vi "Parse Auto Data.vi"(10 "Is Blue Alliance?":bool=TRUE, 11 "path":path) -> (1 "Zero Velocity?":bool[](array[boolean]), 2 "Velocities":T3[](array[typedef]), 3 "Positions":cluster{"x":dbl, "y":dbl, "th":dbl}[](array[cluster]), 5 "Commands out":cluster{"Time (s)":dbl, T1, bool}[](array[cluster]), 7 "Overall":cluster{"Time (s)":dbl, "Distance (ft)":dbl})   [LabVIEW 2023]
uses:
  swerve/Type Definitions/Data/Robot Velocities.ctl
  bordeaux-pathinator/Bordeaux/Types/Single Cmd Info.ctl
  <vilib>/picture/picture.llb/imagedata.ctl
  <vilib>/Analysis/coordinate.llb/2D Cartesian Coordinate Rotation (Scalar).vi
  <vilib>/Analysis/NI_AALPro.lvlib
panel:
  out "XY Graph":cluster{dbl[], dbl[]}[](graph)
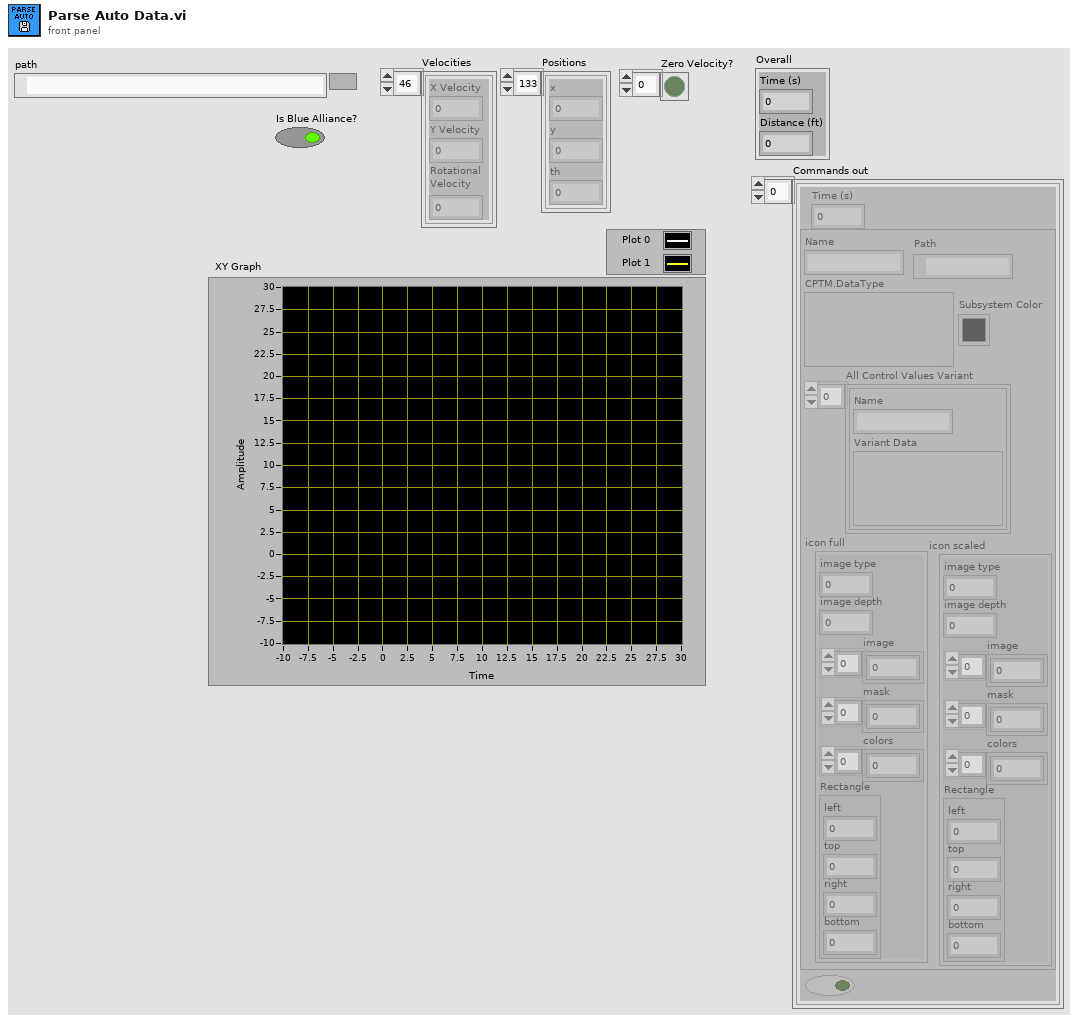
[diagram p1: front panel]
types:
  T1 = typedef "Single Cmd Info.ctl" = cluster{"Name":string, "CPTM.DataType":variant, "All Control Values Variant":cluster{"Name":string, "Variant Data":variant}[], "icon full":T2, "icon scaled":T2, "Path":path, "Subsystem Color":u32}
  T2 = typedef "imagedata.ctl" = cluster{"image type":i32, "image depth":i32, "image":u8[], "mask":u8[], "colors":u32[], "Rectangle":cluster{"left":i16, "top":i16, "right":i16, "bottom":i16}}
  T3 = typedef "Robot Velocities.ctl" = cluster{"X Velocity":dbl, "Y Velocity":dbl, "Rotational \nVelocity":dbl}
  T4 = typedef "Trajectory Data.ctl" = cluster{"Segment Name":string, "Type":T5, "Traj Pos Points":cluster{"x":dbl, "y":dbl, "th":dbl}[], "Traj Vel Points":cluster{"V":dbl, "Omega":dbl, "V vector":cluster{"y":dbl, "x":dbl}}[], "Accel Index":i32, "Decel Index":i32}[]
  T5 = typedef "Segment Type.ctl" = enum16{"Accel Straight", "Const Straight", "Blend", "Circle", "Bezier"}
  T6 = typedef "WPI_DriverStationAllianceInfo.ctl" = enum16{"Red", "Blue", "Invalid"}
  T7 = cluster{"V":dbl, "Omega":dbl, "V vector":cluster{"y":dbl, "x":dbl}}[]
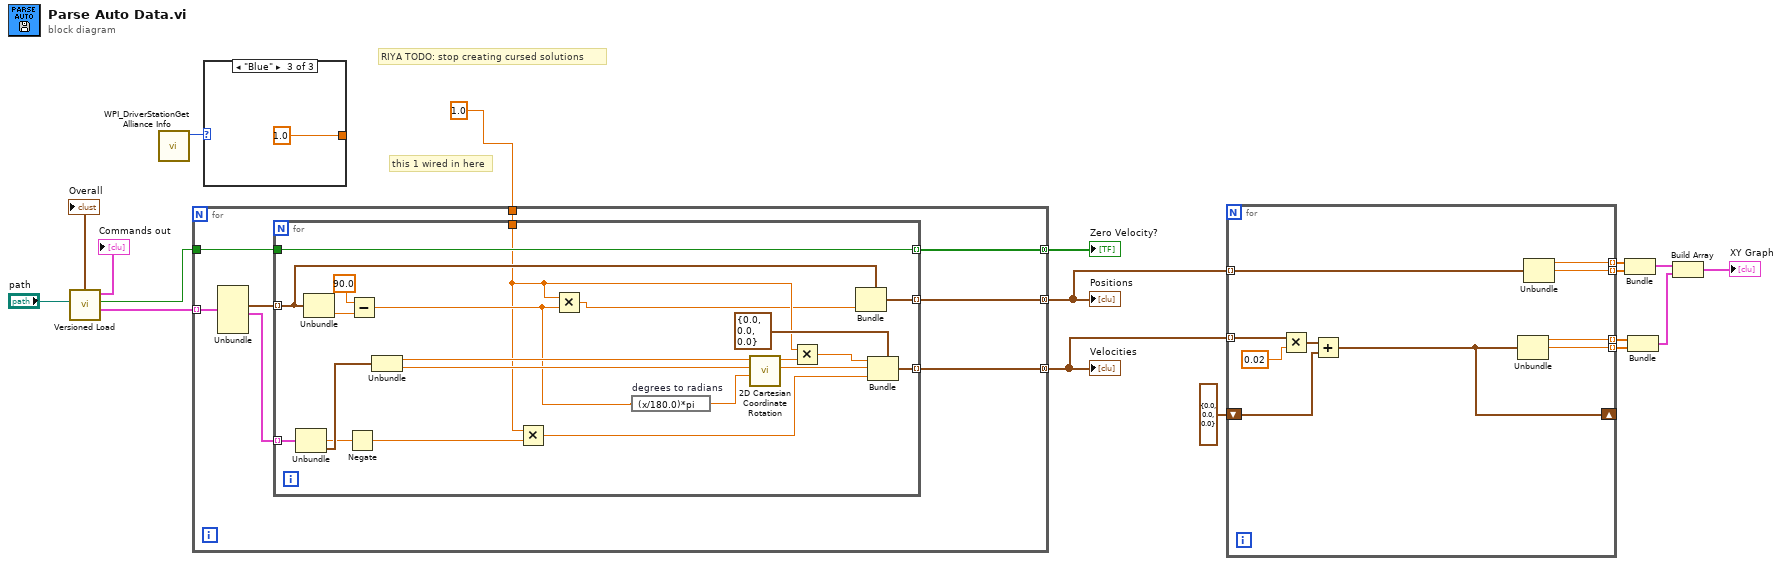
[diagram p0: block diagram]
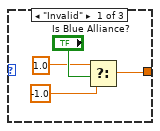
[diagram p2: hidden frame]
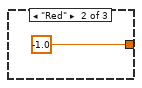
[diagram p3: hidden frame]
diagram:
  # "this 1 wired in here"
  # "RIYA TODO: stop creating cursed solutions"
  n1 = call "Versioned Load.vi"("path"="path") -> ("Trajectory Data"=w18:T4, "Zero V"=w16:bool, "Commands out"=→"Commands out":cluster{"Time (s)":dbl, T1, bool}[], "Overall"=→"Overall":cluster{"Time (s)":dbl, "Distance (ft)":dbl})  [unwired: 3 in, 4 out]
  n2 = call <vilib>:"WPI_DriverStationGet Alliance Info.vi"() -> ("Alliance"=w17:T6)  [unwired: 6 in, 5 out]
  n3 = for {
    tunnel: w18 -> [w26] mode=indexing
    tunnel: [w23] -> w13 mode=concatenating
    tunnel: 1.0 ("f") -> [w22]
    tunnel: [w19] -> w12 mode=concatenating
    tunnel: w16 -> [w21]
    tunnel: [w20] -> w15 mode=concatenating
    n4 = Unbundle(w26) -> ("Traj Pos Points"=w25:cluster{"x":dbl, "y":dbl, "th":dbl}[], "Traj Vel Points"=w24:T7)  [unwired: 4 out]
    n5 = for {
      tunnel: w25 -> [w45] mode=indexing
      tunnel: w24 -> [w43] mode=indexing
      tunnel: [w44] -> w23 mode=indexing
      tunnel: w22 -> [w28]
      tunnel: [w35] -> w19 mode=indexing
      tunnel: w21 -> [w32]
      tunnel: [w32] -> w20 mode=indexing
      n6 = Unbundle(w43) -> ("Omega"=w31:dbl, "V vector"=w42:cluster{"y":dbl, "x":dbl})  [unwired: 1 out]
      n7 = Unbundle(w45) -> ("th"=w47:dbl)  [unwired: 2 out]
      n8 = Negate(x=w31) -> (-x=w30:dbl)
      n9 = Subtract(x=90.0, y=w47) -> (x-y=w29:dbl)
      n10 = Unbundle(w42) -> ("y"=w40:dbl, "x"=w39:dbl)
      n11 = Multiply(x=w28, y=w30) -> (x*y=w37:dbl)
      n12 = Multiply(x=w28, y=w29) -> (x*y=w27:dbl)
      n13 = expression code="(x/180.0)*pi" "degrees to radians"(w29) -> (w41:dbl)
      n14 = call-poly <vilib>:"2D Cartesian Coordinate Rotation.vi"("theta"=w41, "y"=w39, "x"=w40) -> ("y out"=w38:dbl, "x out"=w34:dbl)  [unwired: 6 in, 1 out]
      n15 = Multiply(x=w28, y=w34) -> (x*y=w33:dbl)
      n16 = Bundle(cluster=w45, "th"=w27) -> (w44:cluster{"x":dbl, "y":dbl, "th":dbl})  [unwired: 2 in]
      n17 = Bundle(cluster=T3 {"X Velocity"=0.0, "Y Velocity"=0.0, "Rotational \nVelocity"=0.0} ("Robot Velocities"), "X Velocity"=w33, "Y Velocity"=w38, "Rotational \nVelocity"=w37) -> (w35:T3)
    }
  }
  "Positions" <- w13
  "Velocities" <- w12
  "Zero Velocity?" <- w15
  n18 = case shown="\"Blue\"" w17 {
    tunnel: [w48 -1.0 1.0] -> _
    frame "Invalid" {
      n19 = Select(t=1.0, s="Is Blue Alliance?", f=-1.0) -> (s? t:f=w48:dbl)
    }
    frame "Red" {
    }
    frame "Blue" {
    }
  }
  n20 = for {
    tunnel: w13 -> [w63] mode=indexing
    tunnel: w12 -> [w60] mode=indexing
    tunnel: [w62] -> w11 mode=indexing
    tunnel: [w61] -> w10 mode=indexing
    shift-right: [w56] -> _
    shift-left: T3 {"X Velocity"=0.0, "Y Velocity"=0.0, "Rotational \nVelocity"=0.0} ("Robot Velocities") -> [w57]
    tunnel: [w55] -> w8 mode=indexing
    tunnel: [w54] -> w7 mode=indexing
    n21 = Multiply(x=w60, y=0.02) -> (x*y=w58:T3)
    n22 = Add(x=w58, y=w57) -> (x+y=w56:T3)
    n23 = Unbundle(w56) -> ("X Velocity"=w55:dbl, "Y Velocity"=w54:dbl)  [unwired: 1 out]
    n24 = Unbundle(w63) -> ("x"=w62:dbl, "y"=w61:dbl)  [unwired: 1 out]
  }
  n25 = Bundle(w11, w10) -> (w6:cluster{dbl[], dbl[]})  [unwired: 1 in]
  n26 = Bundle(w8, w7) -> (w5:cluster{dbl[], dbl[]})  [unwired: 1 in]
  n27 = Build Array(w6, w5) -> (→"XY Graph":cluster{dbl[], dbl[]}[])
